vi "Write JSON to Config.vi"(8 "error in (no error)":errorcluster, 10 "JSON String":string, 11 "Plugin Name":string) -> (0 "error out":errorcluster)   [LabVIEW 2021, in "CIFLogs.lvlib"]
uses:
  CIFLogs.lvlib
  Typedef/Message Type.ctl
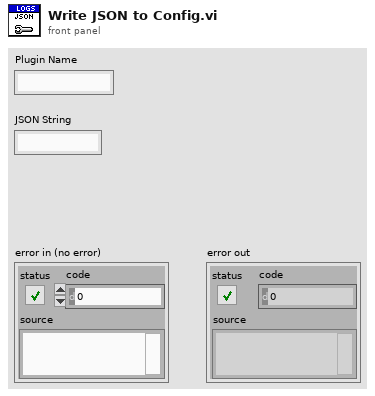
[diagram p1: front panel]
types:
  T1 = typedef "CIFLogs.lvlib/Message Type.ctl" = enum16{"Error", "Information", "Print Terminal", "Configuration"}
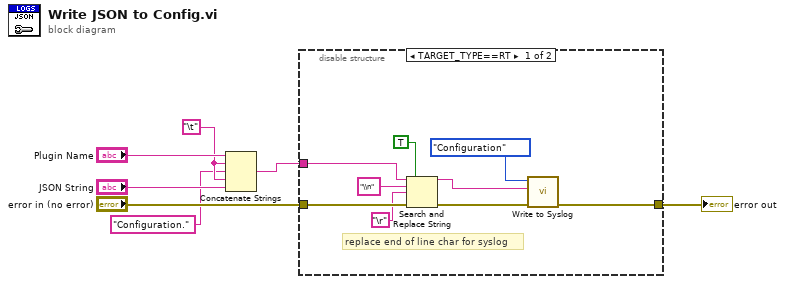
[diagram p0: block diagram]
diagram:
  w2 = "\t"
  n1 = Concatenate Strings("Plugin Name", w2, "Configuration." ("string"), w2, "JSON String") -> (w4:string)
  n2 = disable-structure shown="TARGET_TYPE==RT" {
    disable-tunnel: "error in (no error)" -> [w12 _]
    disable-tunnel: [w16 _] -> w6
    disable-tunnel: w4 -> [w11 _]
    frame condition #0 (active) {
      # "replace end of line char for syslog"
      n3 = Search and Replace String(replace all?=TRUE ("replace all? (F)"), input string=w11, search string="\\n", replace string="\r", error in=w12) -> (result string=w9:string, error out=w10:errorcluster)  [unwired: 3 in, 2 out]
      n4 = call "Write to Syslog.vi"("error in (no error)"=w10, "message"=w9, "CIF Message Type"=Message_Type."Configuration") -> ("error out"=w16:errorcluster)  [unwired: 8 in]
    }
    frame condition #1 {
    }
  }
  "error out" <- w6
